vi "Finish.vi"   [LabVIEW 2017]
doc: "This VI is called just before exiting. It is expected to close I/O refnum, save collected data, etc."
uses:
  <vilib>/Rock Robotics/WPI/Utilities/WPI_GetSetVariantRefNum.vi
  <vilib>/Rock Robotics/WPI/ThirdParty/Sensors/navX/_TypeDefs/FRIC_navX_DeviceNumbersTypeDef.ctl
  <vilib>/Rock Robotics/WPI/Ultrasonic/WPI_SonarMB1010AnalogRefNum Registry Get.vi
  <vilib>/Rock Robotics/WPI/Ultrasonic/WPI_SonarMB1010AnalogClose.vi
panel:
  # "I don't know how to close the navex"
types:
  T1 = typedef "WPI_SonarMB1010AnalogDeviceRef.ctl" = cluster{"AIDeviceRef":T2, "Scaling factor (V/in)":dbl, "Average Bits":u8}
  T2 = typedef "WPI_AnalogChannelDevRef.ctl" = cluster{"DevStatus":errorcluster, "Analog Channel":T3}
  T3 = typedef "FPGA_AIChannel.ctl" = enum8{"AI 0", "AI 1", "AI 2", "AI 3", "AI MXP 0", "AI MXP 1", "AI MXP 2", "AI MXP 3", "Invalid"}
  T4 = typedef "WPI_MotorControlDeviceRef.ctl" = cluster{"DeviceStatus":errorcluster, "Type":T5, "PWM":cluster{"PWM Channel":T6, "DeadBand":T7}, "CAN":cluster{"Device Number":u8, "SetOutput VI Ref":variant, "GetOutput VI Ref":variant, "Enable VI Ref":variant, "Disable VI Ref":variant, "Data":variant}, "Invert":bool, "DIO PWM":cluster{"PWM \"Enable\" Channel":T6, "DIOChannel":T8, "PWM Rate":dbl}}
  T5 = typedef "WPI_MotorControlType.ctl" = enum16{"PWM", "CAN", "DIO PWM"}
  T6 = typedef "FPGA_DIOPWMChannel.ctl" = enum8{"PWM 0", "PWM 1", "PWM 2", "PWM 3", "PWM 4", "PWM 5", "PWM 6", "PWM 7", "PWM 8", "PWM 9", "PWM MXP 0", "PWM MXP 1", "PWM MXP 2", "PWM MXP 3", "PWM MXP 4", "PWM MXP 5", "PWM MXP 6", "PWM MXP 7", "PWM MXP 8", "PWM MXP 9", "Invalid"}
  T7 = typedef "WPI_PWMDeadband.ctl" = cluster{"Name":string, "maxPositivePwm":i32, "minPositivePwm":i32, "centerPwm":i32, "maxNegativePwm":i32, "minNegativePwm":i32, "angularRange":u16}
  T8 = typedef "FPGA_DIOChannel.ctl" = enum8{"DIO 0", "DIO 1", "DIO 2", "DIO 3", "DIO 4", "DIO 5", "DIO 6", "DIO 7", "DIO 8", "DIO 9", "DIO MXP 0", "DIO MXP 1", "DIO MXP 2", "DIO MXP 3", "DIO MXP 4", "DIO MXP 5", "DIO MXP 6", "DIO MXP 7", "DIO MXP 8", "DIO MXP 9", "DIO MXP 10", "DIO MXP 11", "DIO MXP 12", "DIO MXP 13", "DIO MXP 14", "DIO MXP 15", "SPI Port CS1", "SPI Port CS2", "SPI Port CS3", "SPI Port MISO", "SPI Port MOSI", "Invalid"}
  T9 = typedef "WPI_RobotDriveDevRef.ctl" = cluster{"DevStatus":errorcluster, "Motors[]":T4[], "Square Inputs":bool, "Max Output":dbl}
  T10 = typedef "WPI_CompressorDevRef.ctl" = cluster{"DevStatus":errorcluster, "Pneumatics Control Module":u8}
  T11 = typedef "WPI_JoystickDevRef.ctl" = cluster{"Device":T12}
  T12 = typedef "WPI_JoystickDeviceEnum.ctl" = enum16{"USB 0", "USB 1", "USB 2", "USB 3", "USB 4", "USB 5"}
  T13 = typedef "WPI_SolenoidDevRef.ctl" = cluster{"DevStatus":errorcluster, "Pneumatics Control Module":u8, "Forward Solenoid Channel":T14, "Reverse Solenoid Channel":T14}
  T14 = typedef "WPI_SolenoidChannel.ctl" = enum8{"Solenoid 0", "Solenoid 1", "Solenoid 2", "Solenoid 3", "Solenoid 4", "Solenoid 5", "Solenoid 6", "Solenoid 7", "Invalid"}
  T15 = typedef "DriveMotors.ctl" = cluster{"MotorControlDevRef":T4, "MotorControlDevRef":T4, "MotorControlDevRef":T4, "MotorControlDevRef":T4, "MotorControlDevRef":T4, "MotorControlDevRef":T4}
  T16 = typedef "FRIC_navX_DeviceNumbersTypeDef.ctl" = enum16{"Dev0", "Dev1", "Dev2", "Dev3"}
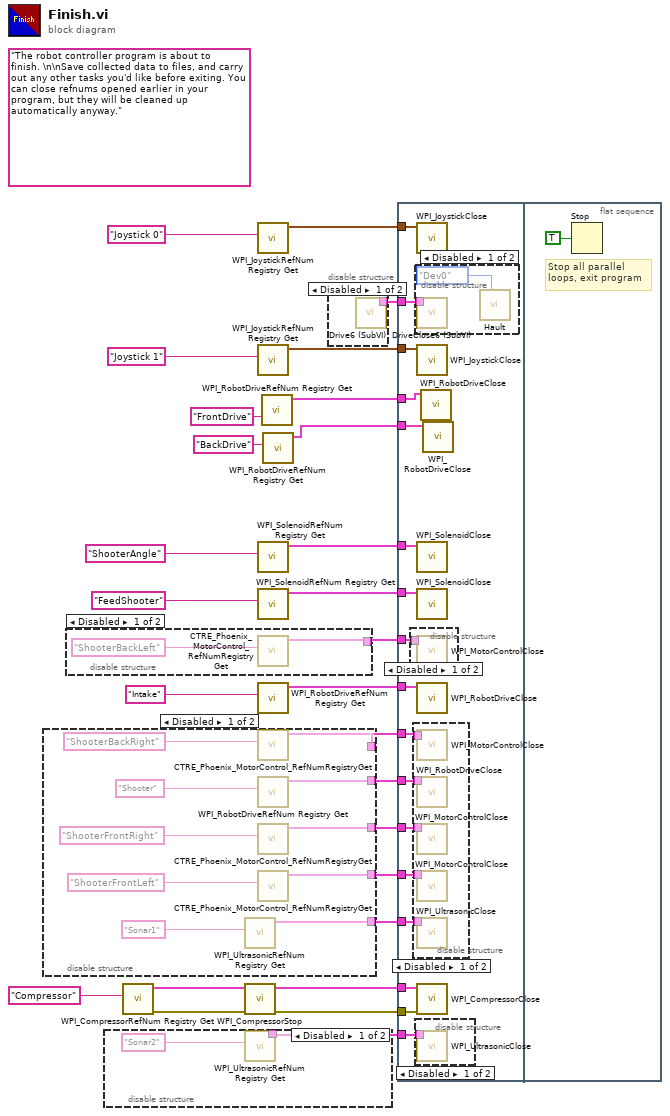
[diagram p0: block diagram]
diagram:
  (unwired) "The robot controller program is about to finish. \n\nSave collected data to files, and carry out any other tasks you'd like before exiting. You can close refnums opened earlier in your program, but they will be cleaned up automatically anyway."
  n1 = disable-structure shown="Disabled" {
    disable-tunnel: [w34 _] -> w25
    disable-tunnel: [w33 _] -> w24
    disable-tunnel: [w32 _] -> w23
    disable-tunnel: [w30 _] -> w16
    disable-tunnel: [w28 _] -> w7
    frame Disabled {
      n2 = call-poly <vilib>:"WPI_UltrasonicRefNum Registry Get.vi"("refnum name"="Sonar1") -> ("SonarMB1010AnalogDevRef"=w28:T1)  [unwired: 9 in, 1 out]
      n3 = call <vilib>:"CTRE_Phoenix_MotorControl_RefNumRegistryGet.vi"("refnum name"="ShooterBackRight") -> ("PhoenixMotorControlDevRef"=w32:T4)  [unwired: 9 in, 1 out]
      n4 = call <vilib>:"WPI_RobotDriveRefNum Registry Get.vi"("refnum name"="Shooter") -> ("RobotDriveDevRef"=w30:T9)  [unwired: 9 in, 1 out]
      n5 = call <vilib>:"CTRE_Phoenix_MotorControl_RefNumRegistryGet.vi"("refnum name"="ShooterFrontRight") -> ("PhoenixMotorControlDevRef"=w33:T4)  [unwired: 9 in, 1 out]
      n6 = call <vilib>:"CTRE_Phoenix_MotorControl_RefNumRegistryGet.vi"("refnum name"="ShooterFrontLeft") -> ("PhoenixMotorControlDevRef"=w34:T4)  [unwired: 9 in, 1 out]
    }
    frame Enabled {
    }
  }
  n7 = disable-structure shown="Disabled" {
    disable-tunnel: [w38 _] -> w22
    frame Disabled {
      n8 = call <vilib>:"CTRE_Phoenix_MotorControl_RefNumRegistryGet.vi"("refnum name"="ShooterBackLeft") -> ("PhoenixMotorControlDevRef"=w38:T4)  [unwired: 9 in, 1 out]
    }
    frame Enabled {
    }
  }
  n9 = disable-structure shown="Disabled" {
    disable-tunnel: [w40 _] -> w6
    frame Disabled {
      n10 = call-poly <vilib>:"WPI_UltrasonicRefNum Registry Get.vi"("refnum name"="Sonar2") -> ("SonarMB1010AnalogDevRef"=w40:T1)  [unwired: 9 in, 1 out]
    }
    frame Enabled {
    }
  }
  n11 = call <vilib>:"WPI_CompressorRefNum Registry Get.vi"("refnum name"="Compressor") -> ("error out"=w12:errorcluster, "CompressorDevRef"=w11:T10)  [unwired: 9 in]
  n12 = call <vilib>:"WPI_CompressorStop.vi"("error in (no error)"=w12, "CompressorDevRef"=w11) -> ("error out"=w10:errorcluster, "CompressorDevRef"=w9:T10)  [unwired: 8 in]
  n13 = call <vilib>:"WPI_JoystickRefNum Registry Get.vi"("refnum name"="Joystick 0") -> ("JoystickDevRef"=w26:T11)  [unwired: 1 in, 9 out]
  n14 = call <vilib>:"WPI_JoystickRefNum Registry Get.vi"("refnum name"="Joystick 1") -> ("JoystickDevRef"=w18:T11)  [unwired: 1 in, 9 out]
  n15 = call <vilib>:"WPI_SolenoidRefNum Registry Get.vi"("refnum name"="ShooterAngle") -> ("SolenoidDevRef"=w19:T13)  [unwired: 9 in, 1 out]
  n16 = call <vilib>:"WPI_SolenoidRefNum Registry Get.vi"("refnum name"="FeedShooter") -> ("SolenoidDevRef"=w13:T13)  [unwired: 9 in, 1 out]
  n17 = call <vilib>:"WPI_RobotDriveRefNum Registry Get.vi"("refnum name"="Intake") -> ("RobotDriveDevRef"=w15:T9)  [unwired: 9 in, 1 out]
  n18 = call <vilib>:"WPI_RobotDriveRefNum Registry Get.vi"("refnum name"="FrontDrive") -> ("RobotDriveDevRef"=w3:T9)  [unwired: 9 in, 1 out]
  n19 = call <vilib>:"WPI_RobotDriveRefNum Registry Get.vi"("refnum name"="BackDrive") -> ("RobotDriveDevRef"=w2:T9)  [unwired: 9 in, 1 out]
  n20 = disable-structure shown="Disabled" {
    disable-tunnel: [w42 _] -> w21
    frame Disabled {
      n21 = call "Drive6 (SubVI).vi"() -> ("DriveControlDevRef"=w42:T15)  [unwired: 11 in]
    }
    frame Enabled {
    }
  }
  n22 = flat-sequence {
    tunnel: w26 -> [w59]
    tunnel: w25 -> [w58]
    tunnel: w24 -> [w57]
    tunnel: w23 -> [w56]
    tunnel: w22 -> [w55]
    tunnel: w21 -> [w54]
    tunnel: w19 -> [w53]
    tunnel: w18 -> [w52]
    tunnel: w16 -> [w51]
    tunnel: w15 -> [w50]
    tunnel: w13 -> [w49]
    tunnel: w10 -> [w48]
    tunnel: w9 -> [w47]
    tunnel: w7 -> [w46]
    tunnel: w6 -> [w45]
    tunnel: w3 -> [w44]
    tunnel: w2 -> [w43]
    frame #0 {
      n23 = disable-structure shown="Disabled" {
        disable-tunnel: w55 -> [w68 _]
        frame Disabled {
          n24 = call <vilib>:"WPI_MotorControlClose.vi"("MotorControlDevRef"=w68) -> ()  [unwired: 10 in, 1 out]
        }
        frame Enabled {
        }
      }
      n25 = disable-structure shown="Disabled" {
        disable-tunnel: w58 -> [w67 _]
        disable-tunnel: w57 -> [w66 _]
        disable-tunnel: w56 -> [w65 _]
        disable-tunnel: w51 -> [w64 _]
        disable-tunnel: w46 -> [w63 _]
        frame Disabled {
          n26 = call <vilib>:"WPI_MotorControlClose.vi"("MotorControlDevRef"=w65) -> ()  [unwired: 10 in, 1 out]
          n27 = call <vilib>:"WPI_RobotDriveClose.vi"("RobotDriveDevRef"=w64) -> ()  [unwired: 10 in, 1 out]
          n28 = call <vilib>:"WPI_MotorControlClose.vi"("MotorControlDevRef"=w66) -> ()  [unwired: 10 in, 1 out]
          n29 = call <vilib>:"WPI_MotorControlClose.vi"("MotorControlDevRef"=w67) -> ()  [unwired: 10 in, 1 out]
          n30 = call-poly <vilib>:"WPI_UltrasonicClose.vi"("SonarMB1010AnalogDevRef"=w63) -> ()  [unwired: 10 in, 1 out]
        }
        frame Enabled {
        }
      }
      n31 = disable-structure shown="Disabled" {
        disable-tunnel: w54 -> [w61 _]
        frame Disabled {
          n32 = call "DriveClose6 (SubVI).vi"("DriveControlDevRef"=w61) -> ()  [unwired: 10 in]
          n33 = call <vilib>:"Hault.vi"("Device Number"=FRIC_navX_DeviceNumbersTypeDef."Dev0") -> ()  [unwired: 11 in]
        }
        frame Enabled {
        }
      }
      n34 = disable-structure shown="Disabled" {
        disable-tunnel: w45 -> [w62 _]
        frame Disabled {
          n35 = call-poly <vilib>:"WPI_UltrasonicClose.vi"("SonarMB1010AnalogDevRef"=w62) -> ()  [unwired: 10 in, 1 out]
        }
        frame Enabled {
        }
      }
      n36 = call <vilib>:"WPI_JoystickClose.vi"("JoystickDevRef"=w59) -> ()  [unwired: 11 out]
      n37 = call <vilib>:"WPI_JoystickClose.vi"("JoystickDevRef"=w52) -> ()  [unwired: 11 out]
      n38 = call <vilib>:"WPI_SolenoidClose.vi"("SolenoidDevRef"=w53) -> ()  [unwired: 10 in, 1 out]
      n39 = call <vilib>:"WPI_SolenoidClose.vi"("SolenoidDevRef"=w49) -> ()  [unwired: 10 in, 1 out]
      n40 = call <vilib>:"WPI_RobotDriveClose.vi"("RobotDriveDevRef"=w50) -> ()  [unwired: 10 in, 1 out]
      n41 = call <vilib>:"WPI_CompressorClose.vi"("error in (no error)"=w48, "CompressorDevRef"=w47) -> ()  [unwired: 9 in, 1 out]
      n42 = call <vilib>:"WPI_RobotDriveClose.vi"("RobotDriveDevRef"=w44) -> ()  [unwired: 10 in, 1 out]
      n43 = call <vilib>:"WPI_RobotDriveClose.vi"("RobotDriveDevRef"=w43) -> ()  [unwired: 10 in, 1 out]
    }
    frame #1 {
      # "Stop all parallel\nloops, exit program"
      n44 = Stop(stop? (T)=TRUE ("Quit")) -> ()
    }
  }
